vi "Main.RTM.AddSinglePointChannels.vi"(8 "error in (no error)":errorcluster, 11 "Node Ptr":u64 format="%.0x") -> (0 "error out":errorcluster)   [LabVIEW 2015]
uses:
  NationalInstruments.VeriStand.SystemStorage
  <vilib>/NI VeriStand/Custom Device API/Custom Device API.lvlib
  <vilib>/NI VeriStand/UI Controls/System Definition Tree/NI_VS UI System Tree.lvlib
  NationalInstruments.VeriStand.SystemStorageUI
  Shared/Single Point/SinglePoint.lvlib
panel:
  in  "OK Button":bool
  in  "TreeBrowserWF":refnum<k24>(container)
  in  "Tag":string
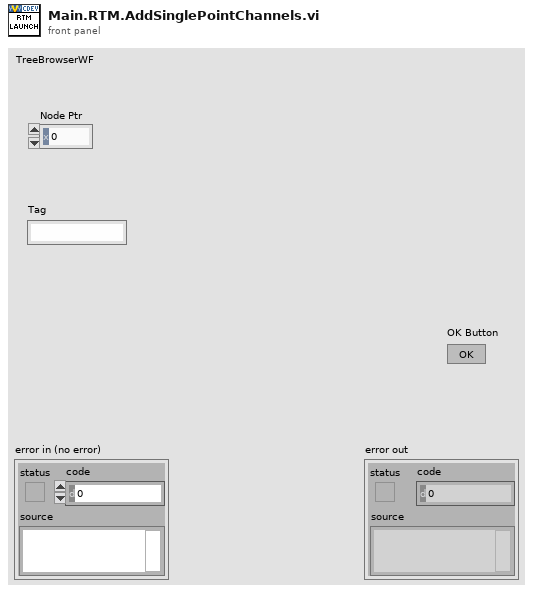
[diagram p1: front panel]
types:
  T1 = typedef "Custom Device API.lvlib/Custom Device Pointer.ctl" = refnum<k24>
  T2 = typedef "NI_VS UI System Tree.lvlib/Callback Type.ctl" = cluster{"Net Callbacks":refnum<k27>[], "Event":T3}
  T3 = typedef "NI_VS UI System Tree.lvlib/Net Event Data Ref.ctl" = refnum<user-event>
  T4 = typedef "NI_VS UI System Tree.lvlib/System Definition Tree Ref.ctl" = refnum<k24>
  T5 = typedef "Custom Device API.lvlib/Custom Device Item Ref.ctl" = u64
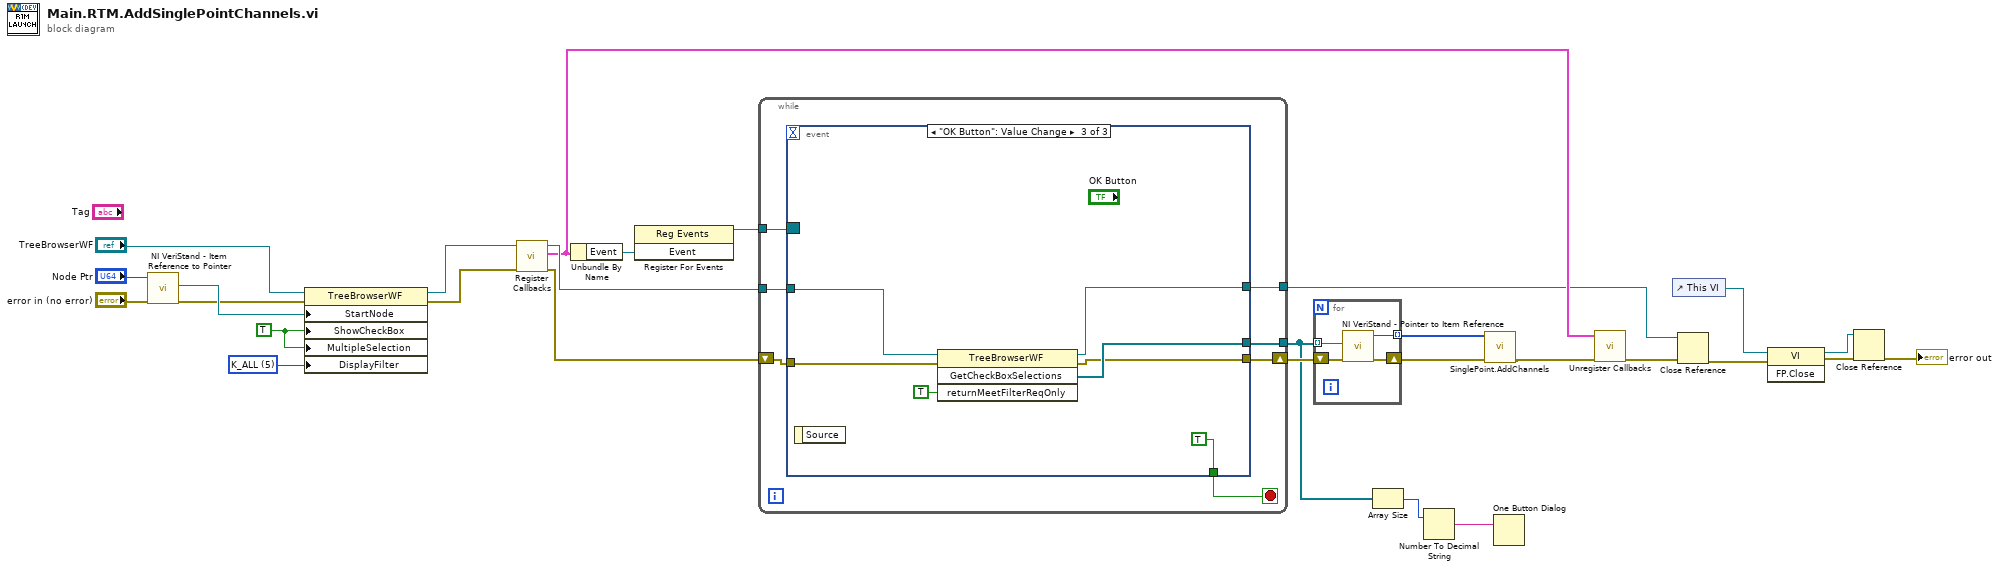
[diagram p0: block diagram]
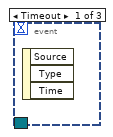
[diagram p2: hidden frame]
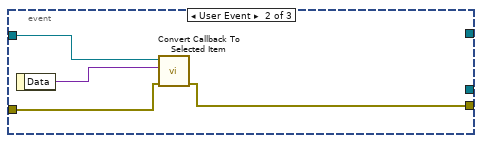
[diagram p3: hidden frame]
diagram:
  w9 = u8 5 items=["K_CHAN_R", "K_CHAN_W", "K_CHAN_RW", "K_CHAN_VOLT", "K_CHAN_FAULT", "K_ALL", "K_CUSTOM", "K_CHAN_R_VIS", "K_CHAN_W_VIS", "K_CHAN_RW_VIS", "K_CHAN_VOLT_VIS", "K_CHAN_FAULT_VIS", "K_WAVE", "K_WAVE_VIS", "K_WAVE_DBL", "K_WAVE_CDB", "K_WAVE_DBL_VIS", "K_WAVE_CDB_VIS"] ("filterType")
  w20 = TRUE ("ShowCheckBox")
  n1 = call <vilib>:"NI VeriStand - Item Reference to Pointer.vi"("error in (no error)"="error in (no error)", "Item Ref in"="Node Ptr") -> ("error out"=w7:errorcluster, "Node Pointer"=w23:T1)  [unwired: 6 in, 2 out]
  n2 = property class="TreeBrowserWF"(reference="TreeBrowserWF", error in=w7, "StartNode"=w23, "ShowCheckBox"=w20, "MultipleSelection"=w20, "DisplayFilter"=w9) -> (reference out=w21:refnum<k24>, error out=w22:errorcluster)
  n3 = call <vilib>:"Register Callbacks.vi"("error in (no error)"=w22, "System Definition Tree"=w21) -> ("error out"=w27:errorcluster, "Callbacks"=w25:T2, "System Definition Tree dup"=w26:T4)  [unwired: 7 in]
  n4 = Unbundle By Name(w25) -> ("Event"=w24:T3)
  n5 = register-events(w24) -> (reference out=w28:refnum<event-registration>)  [unwired: 2 in, 1 out]
  n6 = while {
    tunnel: w28 -> [w35]
    tunnel: w26 -> [w33]
    shift-right: [w32] -> w17
    shift-left: w27 -> [w34]
    tunnel: [w30] -> w16
    tunnel: [w29] -> w6
    stop <- w31 stop-if-true
    n7 = event shown="[2] \"OK Button\": Value Change" {
      selector: w35 -> [_ _ _]
      dyn-events: _ -> [_ _ _]
      timeout: _ -> [_ _ _]
      tunnel: w34 -> [_ w38 w44]
      tunnel: w33 -> [_ w37 w45]
      tunnel: [_ w36 w41] -> w32
      tunnel: [_ _ TRUE] -> w31
      tunnel: [_ _ w43] -> w30
      tunnel: [_ _ w42] -> w29
      event Timeout {
        n8 = event-data() -> ()  [unwired: 1 in, 3 out]
      }
      event User Event {
        n9 = event-data() -> ("Data"=w39:variant)  [unwired: 1 in]
        n10 = call <vilib>:"Convert Callback To Selected Item.vi"("error in"=w38, "Data"=w39, "SystemDefinitionBrowser Ref"=w37) -> ("error out"=w36:errorcluster)  [unwired: 7 in, 1 out]
      }
      event "OK Button": Value Change {
        n11 = event-data() -> ()  [unwired: 1 in, 1 out]
        n12 = invoke class="TreeBrowserWF" method="GetCheckBoxSelections"(reference=w45, error in=w44, "returnMeetFilterReqOnly"=TRUE) -> (reference out=w43:T4, error out=w41:errorcluster, "GetCheckBoxSelections"=w42:refnum<k24>[])  [unwired: 1 in, 1 out]
      }
    }
  }
  n13 = for {
    tunnel: w6 -> [w49] mode=indexing
    tunnel: [w48] -> w3 mode=indexing
    shift-right: [w47] -> w2
    shift-left: w17 -> [w50]
    n14 = call <vilib>:"NI VeriStand - Pointer to Item Reference.vi"("error in (no error)"=w50, "Node Pointer"=w49) -> ("error out"=w47:errorcluster, "Item Ref out"=w48:T5)  [unwired: 8 in]
  }
  n15 = Array Size(array=w6) -> (size(s)=w5:i32)
  n16 = Number To Decimal String(number=w5) -> (decimal integer string=w4:string)  [unwired: 1 in]
  n17 = call "SinglePoint.AddChannels.vi"("Error in"=w2, "Waveform Section Refs"=w3) -> ("Error out"=w1:errorcluster)  [unwired: 9 in]
  n18 = One Button Dialog(message=w4) -> ()  [unwired: 1 in, 1 out]
  n19 = call <vilib>:"Unregister Callbacks.vi"("error in (no error)"=w1, "Callbacks"=w25) -> ("error out"=w15:errorcluster)  [unwired: 9 in]
  n20 = control-ref of="This VI"() -> (w14:refnum<vi>)
  n21 = Close Reference(reference=w16, error in (no error)=w15) -> (error out=w13:errorcluster)
  n22 = invoke class="VI" method="FP.Close"(reference=w14, error in=w13) -> (reference out=w10:refnum<vi>, error out=w12:errorcluster)  [unwired: 1 in, 1 out]
  n23 = Close Reference(reference=w10, error in (no error)=w12) -> (error out=→"error out":errorcluster)
